vi "FormStanMessage.vi"(8 "error in":errorcluster, 10 "data":variant, 11 "Command":string) -> (0 "error out":errorcluster, 3 "message":variant)   [LabVIEW 2015]
uses:
  ControlsVIs/Clusters-def/Standard Command.ctl
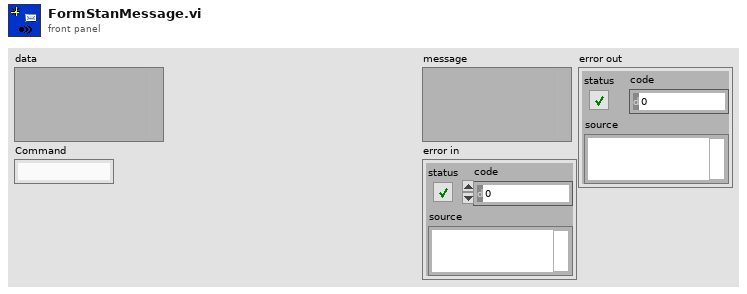
[diagram p1: front panel]
types:
  T1 = typedef "Standard Command.ctl" = cluster{"command":string, "data":variant}
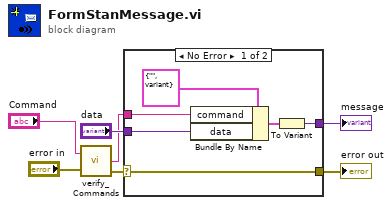
[diagram p0: block diagram]
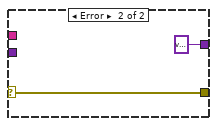
[diagram p2: hidden frame]
diagram:
  n1 = call "verify_Commands.vi"("Command"="Command", "error in"="error in") -> ("Command out"=w4:string, "error out"=w5:errorcluster)  [unwired: 1 out]
  n2 = case shown="No Error" w5 {
    selector: w5 -> [w8 w14]
    tunnel: "data" -> [w11 _]
    tunnel: w4 -> [w10 _]
    tunnel: [w9 variant ("Variant")] -> w3
    tunnel: [w8 w14] -> w2
    frame No Error {
      n3 = Bundle By Name(cluster=T1 {"command"="", "data"=variant} ("input cluster"), "command"=w10, "data"=w11) -> (w12:T1)
      n4 = To Variant(anything=w12) -> (Variant=w9:variant)
    }
    frame Error {
    }
  }
  "message" <- w3
  "error out" <- w2
